vi "Create Listener Refnum.vi"(8 "error in (no error)":errorcluster, 11 "LIBSSH2_LISTENER*":u64 format="%.0x") -> (0 "error out":errorcluster, 3 "listener":T1)   [LabVIEW 2013, in "libssh2.lvlib"]
uses:
  libssh2.lvlib
  Listener Refnum.ctl
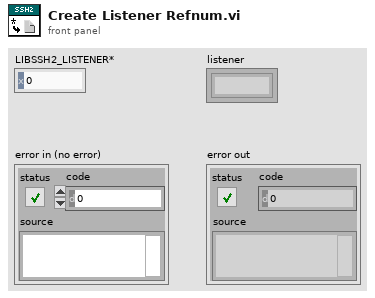
[diagram p1: front panel]
types:
  T1 = typedef "libssh2.lvlib/Listener Refnum.ctl" = refnum<k1>
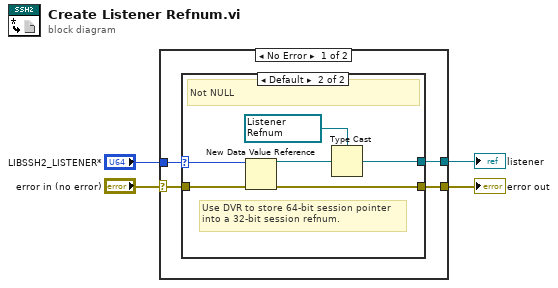
[diagram p0: block diagram]
diagram:
  n1 = case shown="No Error" "error in (no error)" {
    selector: "error in (no error)" -> [w6 w16]
    tunnel: [w8 _] -> w4
    tunnel: "LIBSSH2_LISTENER*" -> [w5 _]
    tunnel: [w7 w16] -> w2
    frame No Error {
      n2 = case shown="Default" w5 {
        selector: w5 -> [_ w10]
        tunnel: [_ w13] -> w8
        tunnel: [w9 w12] -> w7
        tunnel: w6 -> [w9 w11]
        frame 0 {
          # "NULL"
        }
        frame Default {
          w14 = T1 refnum items=["Listener"] ("listener")
          # "Use DVR to store 64-bit session pointer\ninto a 32-bit session refnum."
          # "Not NULL"
          n3 = New Data Value Reference(data value=w10, error in=w11) -> (data value reference=w15:refnum<data-value>, error out=w12:errorcluster)
          n4 = Type Cast(type=w14, x=w15) -> (*(type *) &x=w13:T1)
        }
      }
    }
    frame Error {
    }
  }
  "listener" <- w4
  "error out" <- w2
